vi "Snap to left.vi"(8 "centered? (F)":bool, 9 "Fixed Rect":T1, 11 "Rect":T1) -> (1 "TopLeft point":cluster{"x":i32, "y":i32}, 3 "Snapped to left":T1)   [LabVIEW 2012]
doc: "This VI calculates the position of a snapped-to-left rectangle from the positions of a large rectangle and a smaller one that will be positioned inside."
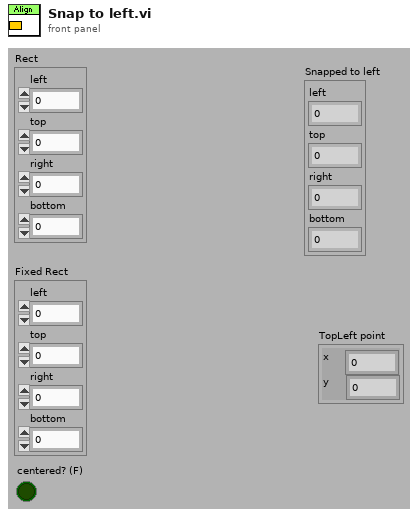
[diagram p1: front panel]
types:
  T1 = cluster{"left":i16, "top":i16, "right":i16, "bottom":i16}
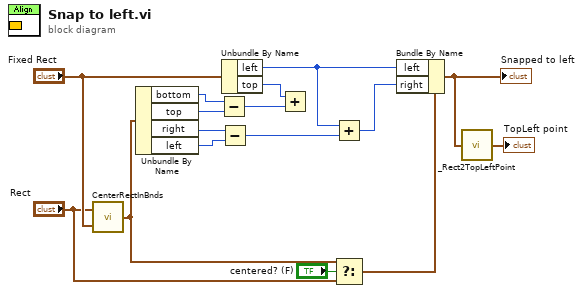
[diagram p0: block diagram]
diagram:
  n1 = call <vilib>:"CenterRectInBnds.vi"("bounds"="Fixed Rect", "rect"="Rect") -> ("centered rect"=w2:T1)
  n2 = Unbundle By Name(w2) -> ("bottom"=w16:i16, "top"=w15:i16, "right"=w11:i16, "left"=w10:i16)
  n3 = Subtract(x=w16, y=w15) -> (x-y=w14:i16)
  n4 = Subtract(x=w11, y=w10) -> (x-y=w8:i16)
  n5 = Unbundle By Name("Fixed Rect") -> ("left"=w9:i16, "top"=w13:i16)
  n6 = Add(x=w13, y=w14) -> ()  [unwired: 1 out]
  n7 = Add(x=w9, y=w8) -> (x+y=w7:i16)
  n8 = Select(t=w2, s="centered? (F)", f="Rect") -> (s? t:f=w3:T1)
  n9 = Bundle By Name(cluster=w3, "left"=w9, "right"=w7) -> (w6:T1)
  "Snapped to left" <- w6
  n10 = call "_Rect2TopLeftPoint.vi"("bounds"=w6) -> ("TopLeft point"=→"TopLeft point":cluster{"x":i32, "y":i32})  [unwired: 4 out]
